vi "stop_sweep.vi"(8 "error in (no error)":errorcluster, 11 "StimulatorDL090727DAQmx in":refnum<class "StimulatorDL090727Writer.lvclass">) -> (0 "error out":errorcluster, 3 "StimulatorDL090727DAQmx out":refnum<class "StimulatorDL090727Writer.lvclass">)   [LabVIEW 2010, in "StimulatorDL090727Writer.lvclass"]
uses:
  StimulatorDL090727Writer.lvclass
  StimulatorDL090724Scaffold/StimulatorDL090724Scaffold/Stimulator090724Scaffold.lvclass
  StimulatorDL090727Writer.lvclass/StimulatorDL090727Writer.ctl
  SignalWriter/GenericSignalWriter/GenericSignalWriter/GenericSignalWriter.lvclass
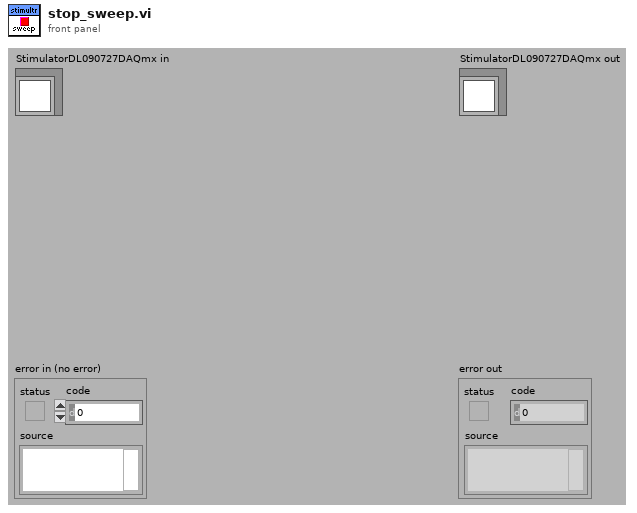
[diagram p1: front panel]
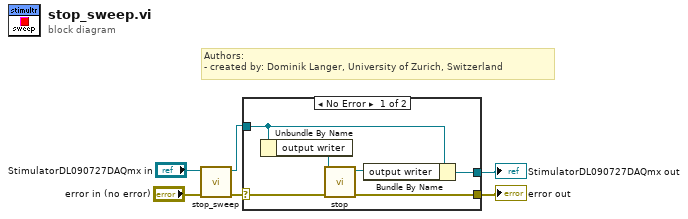
[diagram p0: block diagram]
diagram:
  # "Authors: \n- created by: Dominik Langer, University of Zurich, Switzerland"
  n1 = call-parent "stop_sweep.vi"("error in (no error)"="error in (no error)", "Stimulator090724Scaffold in"="StimulatorDL090727DAQmx in") -> ("error out"=w3:errorcluster, "Stimulator090724Scaffold out"=w1:refnum<class "StimulatorDL090727Writer.lvclass">)  [unwired: 8 in]
  n2 = case shown="No Error" w3 {
    selector: w3 -> [w8 w14]
    tunnel: [w7 w14] -> w6
    tunnel: [w9 w13] -> w5
    tunnel: w1 -> [w10 w13]
    frame No Error {
      n3 = Unbundle By Name(w10) -> ("output writer"=w12:refnum<class "GenericSignalWriter.lvclass">)
      n4 = call-dynamic "stop.vi"("error in (no error)"=w8, "WriteSignalsGenericPlugin in"=w12) -> ("error out"=w7:errorcluster, "WriteSignalsGenericPlugin out"=w11:refnum<class "GenericSignalWriter.lvclass">)  [unwired: 8 out]
      n5 = Bundle By Name(cluster=w10, "output writer"=w11) -> (w9:refnum<class "StimulatorDL090727Writer.lvclass">)
    }
    frame Error {
    }
  }
  "error out" <- w6
  "StimulatorDL090727DAQmx out" <- w5
